vi "Get MyComputer.vi"(8 "error in (no error)":errorcluster, 11 "Project in":refnum<vi>) -> (0 "error out":errorcluster, 2 "My Computer":refnum<vi>, 3 "Project out":refnum<vi>)   [LabVIEW 2019, in "gRPC Scripting Tools.lvlib"]
uses:
  gRPC Scripting Tools.lvlib
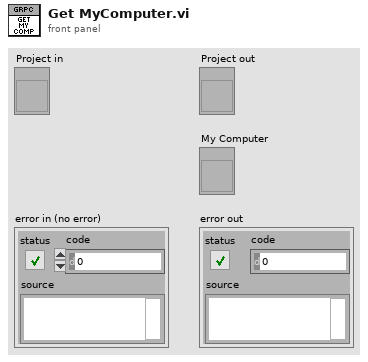
[diagram p1: front panel]
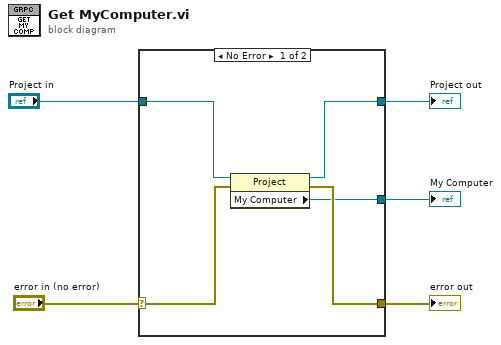
[diagram p0: block diagram]
diagram:
  n1 = case shown="No Error" "error in (no error)" {
    selector: "error in (no error)" -> [w6 w11]
    tunnel: [w10 w12] -> w5
    tunnel: [w9 w11] -> w4
    tunnel: [w8 _] -> w3
    tunnel: "Project in" -> [w7 w12]
    frame No Error {
      n2 = property class="Project"(reference=w7, error in=w6) -> (reference out=w10:refnum<vi>, error out=w9:errorcluster, "My Computer"=w8:refnum<vi>)
    }
    frame Error {
    }
  }
  "Project out" <- w5
  "error out" <- w4
  "My Computer" <- w3
